vi "Position Boundary.vi"(10 "NxN":i32, 11 "Accident Position":T1) -> (3 "In Range?":bool)   [LabVIEW 2015]
uses:
  Data Def/Accident Position.ctl
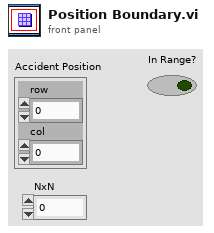
[diagram p1: front panel]
types:
  T1 = typedef "Accident Position.ctl" = cluster{"row":i32, "col":i32}
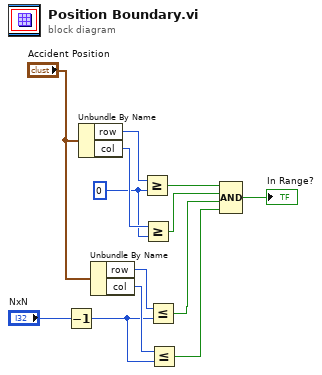
[diagram p0: block diagram]
diagram:
  w11 = 0 ("y")
  n1 = Decrement(x="NxN") -> (x-1=w6:i32)
  n2 = Unbundle By Name("Accident Position") -> ("row"=w13:i32, "col"=w12:i32)
  n3 = Unbundle By Name("Accident Position") -> ("row"=w9:i32, "col"=w7:i32)
  n4 = Greater Or Equal?(x=w13, y=w11) -> (x >= y?=w5:bool)
  n5 = Greater Or Equal?(x=w12, y=w11) -> (x >= y?=w4:bool)
  n6 = Less Or Equal?(x=w9, y=w6) -> (x <= y?=w3:bool)
  n7 = Less Or Equal?(x=w7, y=w6) -> (x <= y?=w2:bool)
  n8 = Compound Arithmetic op=AND(w5, w4, w3, w2) -> (→"In Range?":bool)
